vi "ExecuteGrSimTestPasse.vi"(0 "RandomAllyPoints":dbl[][](array[numeric]), 1 "IA State Input":T3, 3 "Atacando contra?":bool, 5 "id":i32, 9 "reset":bool, 11 "Região do campo\nTeste Passe":enum16{"3", "2", "1", "0", "-1", "-2", "-3"}(ring), 12 "Replace Robots":bool, 14 "Number of Points":i32, 15 "RandomEnemyPoints":dbl[][](array[numeric])) -> (4 "grSim replacement":cluster{"robots":T1[], "ball":T2}={"robots"=[{"x"=0.0, "y"=-450.0, "dir"=0.0, "yellowteam"=FALSE, "id"=0}, {"x"=0.0, "y"=-270.0, "dir"=0.0, "yellowteam"=FALSE, "id"=1}, {"x"=0.0, "y"=-90.0, "dir"=0.0, "yellowteam"=FALSE, "id"=2}, {"x"=0.0, "y"=90.0, "dir"=0.0, "yellowteam"=FALSE, "id"=3}, {"x"=0.0, "y"=270.0, "dir"=0.0, "yellowteam"=FALSE, "id"=4}, {"x"=0.0, "y"=450.0, "dir"=0.0, "yellowteam"=FALSE, "id"=5}], "ball"={"x"=0.0, "y"=0.0, "vx"=0.0, "vy"=0.0}}, 6 "Replace active":bool, 8 "Number of goals":i16, 10 "kick num":i32)   [LabVIEW 2017]
uses:
  Core/AI Input.ctl
  Core/AI Robot.ctl
  Intel/Functions Enum.ctl
  Intel/AttackerStates.ctl
  Path Planning/RRT/PathDests.ctl
  Path Planning/RRT/PathDest.ctl
  Core/AI Ball.ctl
  Core/Field Size.ctl
  Core/AI Judge.ctl
  Intel/Command Enum.ctl
  Util/Events/Events.ctl
  grSim RobotReplacement.ctl
  grSim_BallReplacement.ctl
panel:
  in  "Time":enum16{"Azul", "Amarelo"}(ring) caption="Enum"
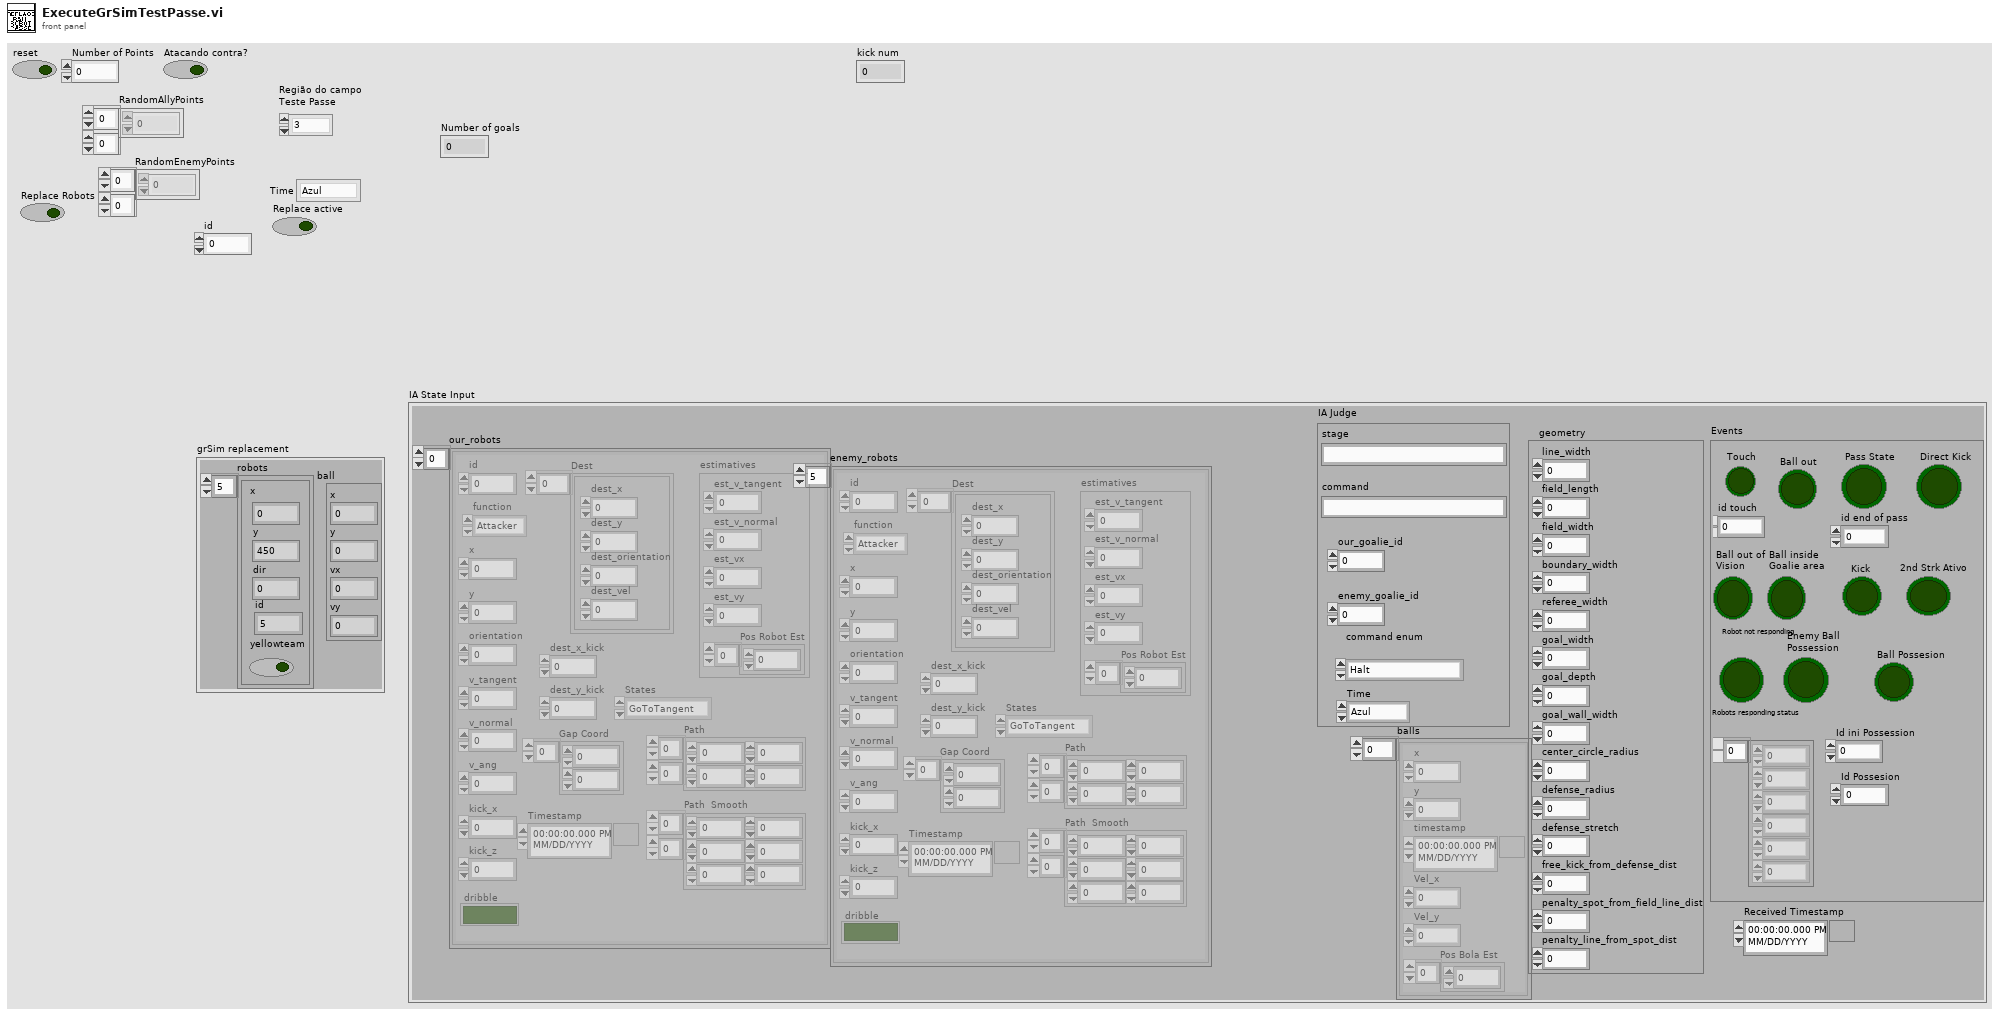
[diagram p1: front panel]
types:
  T1 = typedef "grSim RobotReplacement.ctl" = cluster{"x":dbl, "y":dbl, "dir":dbl, "yellowteam":bool, "id":u32}
  T2 = typedef "grSim_BallReplacement.ctl" = cluster{"x":dbl, "y":dbl, "vx":dbl, "vy":dbl}
  T3 = typedef "AI Input.ctl" = cluster{"our_robots":T4[], "enemy_robots":T4[], "balls":T9[], "geometry":T10, "IA Judge":T11, "Received Timestamp":timestamp, "Events":T13}
  T4 = typedef "AI Robot.ctl" = cluster{"id":u32, "function":T5, "x":dbl, "y":dbl, "orientation":dbl, "v_tangent":dbl, "v_normal":dbl, "v_ang":dbl, "kick_x":dbl, "kick_z":dbl, "dribble":bool, "Timestamp":timestamp, "estimatives":cluster{"est_v_tangent":dbl, "est_v_normal":dbl, "est_vx":dbl, "est_vy":dbl, "Pos Robot Est":dbl[]}, "dest_x_kick":dbl, "dest_y_kick":dbl, "Gap Coord":dbl[], "States":T6, "Path ":dbl[][], "Path  Smooth":dbl[][], "Dest":T7}
  T5 = typedef "Functions Enum.ctl" = enum16{"2nd Striker", "Attacker", "Goalie", "Defender", "Striker", "Goto 0", "Dummy", "Kicker", "ZigZag 0", "ZigZag 1", "ZigZag 2", "ZigZag 3", "ZigZag 4", "ZigZag 5", "ZigZag 6", "ZigZag 7", "ZigZag 8", ""}
  T6 = typedef "AttackerStates.ctl" = enum16{"Pass", "GoToTangent", "BallGetting", "GoToKick", ""}
  T7 = typedef "PathDests.ctl" = T8[]
  T8 = typedef "PathDest.ctl" = cluster{"dest_x":dbl, "dest_y":dbl, "dest_orientation":dbl, "dest_vel":dbl}
  T9 = typedef "AI Ball.ctl" = cluster{"x":dbl, "y":dbl, "timestamp":timestamp, "Vel_x":dbl, "Vel_y":dbl, "Pos Bola Est":dbl[]}
  T10 = typedef "Field Size.ctl" = cluster{"line_width":u32, "field_length":u32, "field_width":u32, "boundary_width":u32, "referee_width":u32, "goal_width":u32, "goal_depth":u32, "goal_wall_width":u32, "center_circle_radius":u32, "defense_radius":u32, "defense_stretch":u32, "free_kick_from_defense_dist":u32, "penalty_spot_from_field_line_dist":u32, "penalty_line_from_spot_dist":u32}
  T11 = typedef "AI Judge.ctl" = cluster{"stage":string, "command":string, "our_goalie_id":dbl, "enemy_goalie_id":dbl, "command enum":T12, "Time":enum16{"Azul", "Amarelo"}}
  T12 = typedef "Command Enum.ctl" = enum16{"Halt", "Stop", "Force Start", "PKA Normal Start", "Prepare Kickoff Ally", "PKE Normal Start", "Prepare Kickoff Enemy", "Prepare Penalty Ally", "PPA Normal Start", "Prepare Penalty Enemy", "PPE Normal Start", "Direct Free Enemy", "Direct Free Ally", "Indirect Free Enemy", "Indirect Free Ally", "Timeout Enemy", "Timeout Ally", "Goal Enemy", "Goal Ally", "Ball Placement Enemy", "Ball Placement Ally", "Normal Half Time", "Extra Time Break", "Extra Half Time", "None", "Post Game"}
  T13 = typedef "Events.ctl" = cluster{"Touch":bool, "Ball out":bool, "id touch":dbl, "Ball out of \nVision":bool, "Ball inside \nGoalie area":bool, "Robot not responding":bool, "Robots responding status":dbl[], "Enemy Ball \nPossession":bool, "Pass State":bool, "id end of pass":dbl, "Kick":bool, "Id ini Possession":dbl, "Ball Possesion":bool, "Id Possesion":dbl, "Direct Kick":bool, "2nd Strk Ativo":bool}
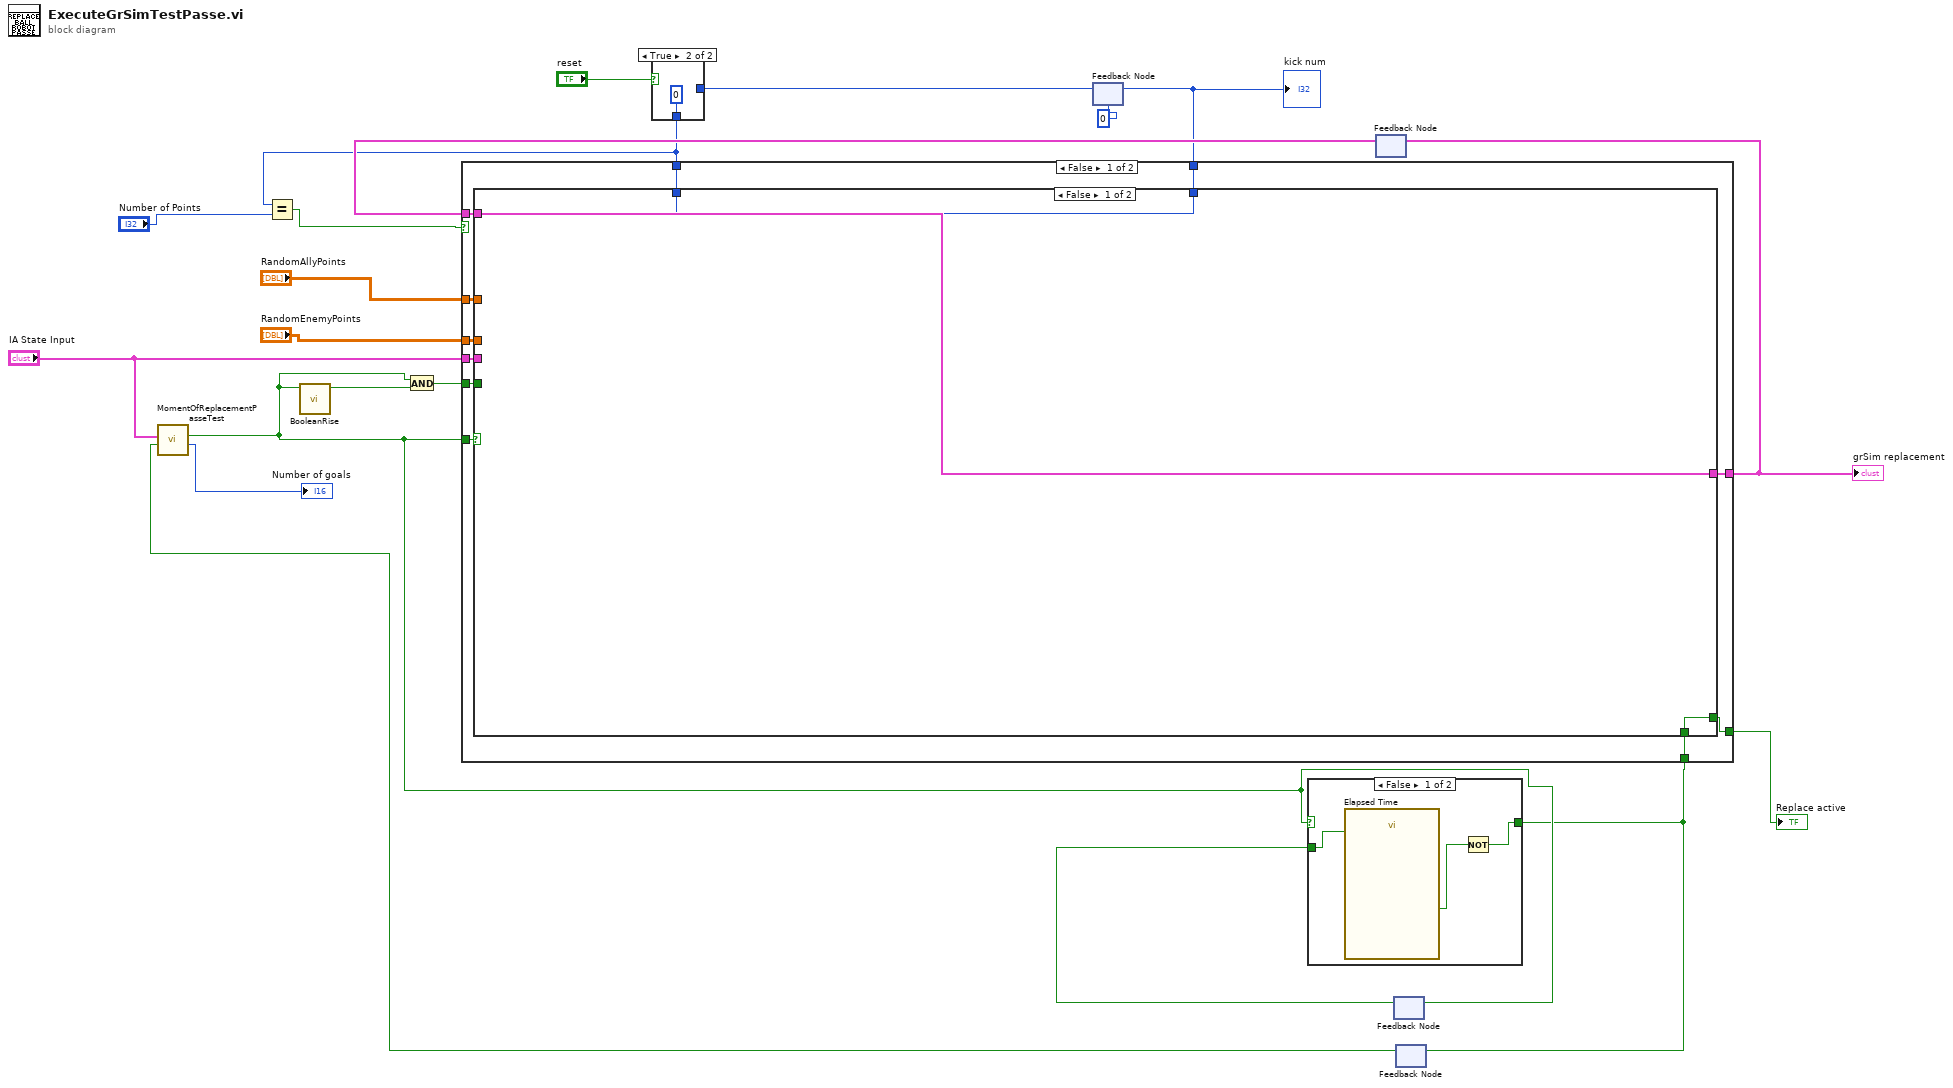
[diagram p0: block diagram]
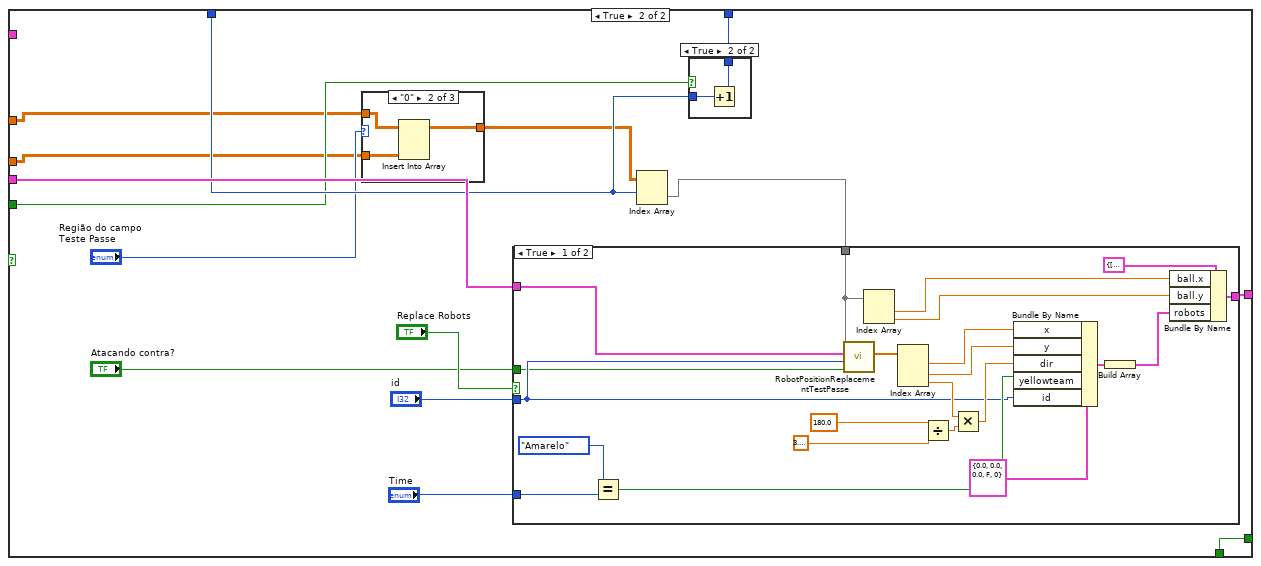
[diagram p2: hidden frame]
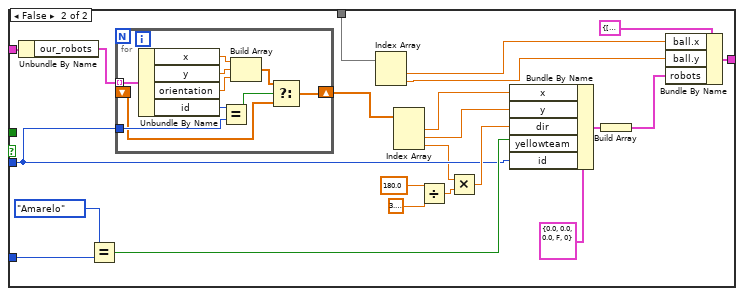
[diagram p6: hidden frame]
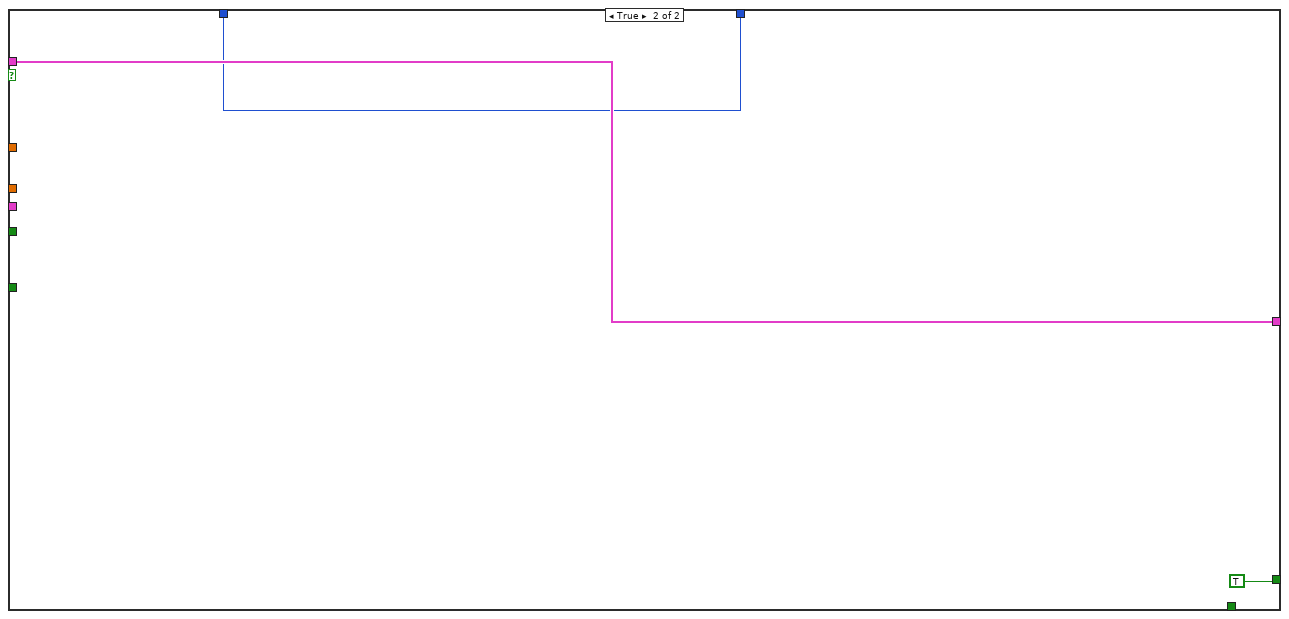
[diagram p7: hidden frame]
diagram:
  n1 = feedback #1(0) -> (w10:i32)
  n2 = case shown="True" "reset" {
    tunnel: w10 -> [w21 _]
    tunnel: [w21 0] -> w7
    frame False {
    }
    frame True {
    }
  }
  n3 = Equal?(x=w7, y="Number of Points") -> (x = y?=w6:bool)
  n4 = feedback #2() -> (w20:cluster{"robots":T1[], "ball":T2})  [unwired: 1 in]
  n5 = feedback #3() -> (w19:bool)  [unwired: 1 in]
  n6 = feedback #4() -> (w16:bool)  [unwired: 1 in]
  n7 = call "MomentOfReplacementPasseTest.vi"("Replace active"=w16, "IA State Input"="IA State Input") -> ("Number of goals"=→"Number of goals":i16, "Time to replace?"=w11:bool)  [unwired: 8 in]
  n8 = call "BooleanRise.vi"("Test Mode On"=w11) -> ("Boolean"=w12:bool)  [unwired: 10 in]
  n9 = And(x=w11, y=w12) -> (x .and. y?=w13:bool)
  n10 = case shown="False" w11 {
    selector: w11 -> [_ w26]
    tunnel: [w25 w26] -> w5
    tunnel: w19 -> [w23 _]
    frame False {
      n11 = call "Elapsed Time"("Reset"=w23) -> ("Time has Elapsed"=w24:bool)  [unwired: 11 in, 7 out]
      n12 = Not(x=w24) -> (.not. x?=w25:bool)
    }
    frame True {
    }
  }
  n13 = case shown="False" w6 {
    tunnel: w20 -> [w37 w119]
    tunnel: [w36 w119] -> w18
    tunnel: "IA State Input" -> [w35 _]
    tunnel: "RandomAllyPoints" -> [w34 _]
    tunnel: [w33 w118] -> w14
    tunnel: w13 -> [w32 _]
    tunnel: w11 -> [w31 _]
    tunnel: w7 -> [w30 w118]
    tunnel: w5 -> [w28 _]
    tunnel: [w29 TRUE] -> w4
    tunnel: "RandomEnemyPoints" -> [w27 _]
    frame False {
      n14 = case shown="False" w31 {
        tunnel: [w40 w55] -> w36
        tunnel: w35 -> [_ w52]
        tunnel: w37 -> [w40 _]
        tunnel: w34 -> [_ w43]
        tunnel: w30 -> [w39 w49]
        tunnel: [w39 w48] -> w33
        tunnel: w32 -> [_ w47]
        tunnel: [w38 w46] -> w29
        tunnel: w28 -> [w38 w46]
        tunnel: w27 -> [_ w42]
        frame False {
        }
        frame True {
          n15 = case shown="\"0\"" "Região do campo\nTeste Passe" {
            tunnel: w43 -> [w56 w59 _]
            tunnel: w42 -> [_ w58 w60]
            tunnel: [w56 w57 w60] -> w41
            frame "-1".."-3" {
            }
            frame "0" {
              n16 = Insert Into Array(array=w59, new element=w58) -> (w57:dbl[][])  [unwired: 2 in]
            }
            frame "3".."1" {
            }
          }
          n17 = Index Array(array=w41, index (row)=w49) -> (element=w54:dbl[])  [unwired: 1 in]
          n18 = case shown="True" "Replace Robots" {
            tunnel: [w85 w107] -> w55
            tunnel: w54 -> [w68 w89]
            tunnel: "Time" -> [w81 w103]
            tunnel: w52 -> [w76 w96]
            tunnel: "id" -> [w69 w94]
            tunnel: "Atacando contra?" -> [w64 _]
            frame True {
              n19 = Equal?(x=enum16{"Azul", "Amarelo"}."Amarelo", y=w81) -> (x = y?=w79:bool)
              n20 = call "RobotPositionReplacementTestPasse.vi"("Atacando contra?"=w64, "id"=w69, "IA State Input"=w76, "Position Ball"=w68) -> ("Position Robot"=w78:dbl[])  [unwired: 5 in]
              n21 = Index Array(array=w68) -> (element #1=w67:dbl, element #2=w66:dbl)  [unwired: 2 in]
              n22 = Index Array(array=w78) -> (element #1=w77:dbl, element #2=w75:dbl, element #3=w70:dbl)  [unwired: 3 in]
              n23 = Divide(x=180.0, y=3.141592653589793) -> (x/y=w73:dbl)
              n24 = Multiply(x=w70, y=w73) -> (x*y=w74:dbl)
              n25 = Bundle By Name(cluster=T1 {"x"=0.0, "y"=0.0, "dir"=0.0, "yellowteam"=FALSE, "id"=0} ("element"), "x"=w77, "y"=w75, "dir"=w74, "yellowteam"=w79, "id"=w69) -> (w83:T1)
              n26 = Build Array(w83) -> (w82:T1[])
              n27 = Bundle By Name(cluster=cluster{"robots":T1[], "ball":T2} {"robots"=[{"x"=0.0, "y"=-450.0, "dir"=0.0, "yellowteam"=FALSE, "id"=0}, {"x"=0.0, "y"=-270.0, "dir"=0.0, "yellowteam"=FALSE, "id"=1}, {"x"=0.0, "y"=-90.0, "dir"=0.0, "yellowteam"=FALSE, "id"=2}, {"x"=0.0, "y"=90.0, "dir"=0.0, "yellowteam"=FALSE, "id"=3}, {"x"=0.0, "y"=270.0, "dir"=0.0, "yellowteam"=FALSE, "id"=4}, {"x"=0.0, "y"=450.0, "dir"=0.0, "yellowteam"=FALSE, "id"=5}], "ball"={"x"=0.0, "y"=0.0, "vx"=0.0, "vy"=0.0}} ("grSim replacement"), "ball.x"=w67, "ball.y"=w66, "robots"=w82) -> (w85:cluster{"robots":T1[], "ball":T2})
            }
            frame False {
              n28 = Unbundle By Name(w96) -> ("our_robots"=w95:T4[])
              n29 = Equal?(x=enum16{"Azul", "Amarelo"}."Amarelo", y=w103) -> (x = y?=w101:bool)
              n30 = for {
                tunnel: w95 -> [w117] mode=indexing
                tunnel: w94 -> [w115]
                shift-right: [w109] -> w93
                shift-left: _ -> [w108]
                n31 = Unbundle By Name(w117) -> ("x"=w114:dbl, "y"=w113:dbl, "orientation"=w112:dbl, "id"=w116:u32)
                n32 = Equal?(x=w116, y=w115) -> (x = y?=w111:bool)
                n33 = Build Array(w114, w113, w112) -> (w110:dbl[])
                n34 = Select(t=w110, s=w111, f=w108) -> (s? t:f=w109:dbl[])
              }
              n35 = Index Array(array=w89) -> (element #1=w88:dbl, element #2=w87:dbl)  [unwired: 2 in]
              n36 = Index Array(array=w93) -> (element #1=w92:dbl, element #2=w90:dbl, element #3=w91:dbl)  [unwired: 3 in]
              n37 = Divide(x=180.0, y=3.141592653589793) -> (x/y=w99:dbl)
              n38 = Multiply(x=w91, y=w99) -> (x*y=w100:dbl)
              n39 = Bundle By Name(cluster=T1 {"x"=0.0, "y"=0.0, "dir"=0.0, "yellowteam"=FALSE, "id"=0} ("element"), "x"=w92, "y"=w90, "dir"=w100, "yellowteam"=w101, "id"=w94) -> (w105:T1)
              n40 = Build Array(w105) -> (w104:T1[])
              n41 = Bundle By Name(cluster=cluster{"robots":T1[], "ball":T2} {"robots"=[{"x"=0.0, "y"=-450.0, "dir"=0.0, "yellowteam"=FALSE, "id"=0}, {"x"=0.0, "y"=-270.0, "dir"=0.0, "yellowteam"=FALSE, "id"=1}, {"x"=0.0, "y"=-90.0, "dir"=0.0, "yellowteam"=FALSE, "id"=2}, {"x"=0.0, "y"=90.0, "dir"=0.0, "yellowteam"=FALSE, "id"=3}, {"x"=0.0, "y"=270.0, "dir"=0.0, "yellowteam"=FALSE, "id"=4}, {"x"=0.0, "y"=450.0, "dir"=0.0, "yellowteam"=FALSE, "id"=5}], "ball"={"x"=0.0, "y"=0.0, "vx"=0.0, "vy"=0.0}} ("grSim replacement"), "ball.x"=w88, "ball.y"=w87, "robots"=w104) -> (w107:cluster{"robots":T1[], "ball":T2})
            }
          }
          n42 = case shown="True" w47 {
            tunnel: w49 -> [w61 w63]
            tunnel: [w61 w62] -> w48
            frame False {
            }
            frame True {
              n43 = Increment(x=w63) -> (x+1=w62:i32)
            }
          }
        }
      }
    }
    frame True {
    }
  }
  "grSim replacement" <- w18
  "Replace active" <- w4
  "kick num" <- w14
  n44 = feedback-in #1(w14) -> ()
  n45 = feedback-in #2(w18) -> ()
  n46 = feedback-in #3(w11) -> ()
  n47 = feedback-in #4(w5) -> ()
